vi "CMN_2DArr2Str.vi"(9 "separator":string=" ", 10 "array in":string[][](table)) -> (2 "string out":string)   [LabVIEW 2016]
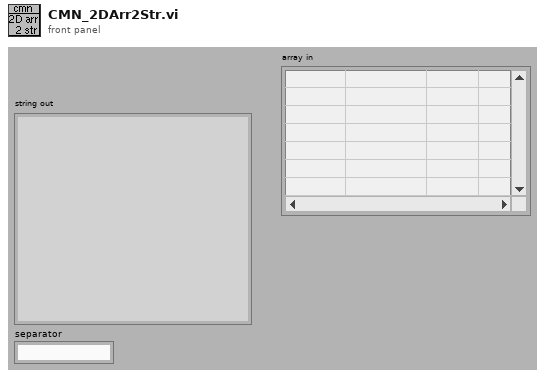
[diagram p1: front panel]
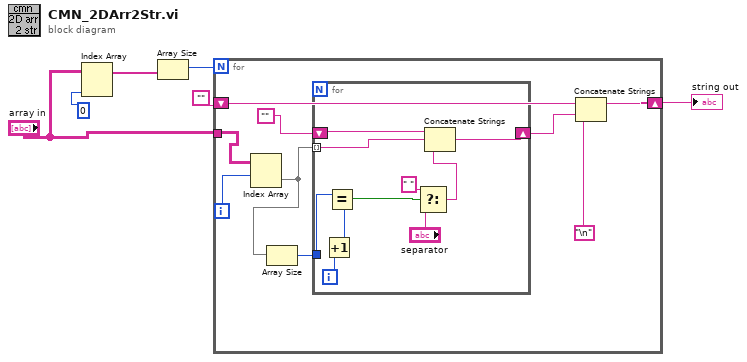
[diagram p0: block diagram]
diagram:
  n1 = Index Array(array="array in", index (col)=0) -> (element=w4:string[])  [unwired: 1 in]
  n2 = Array Size(array=w4) -> (size(s)=w2:i32)
  n3 = for {
    N: w2 -> [_]
    shift-right: [w15] -> w5
    shift-left: "" -> [w14]
    tunnel: "array in" -> [w11]
    i -> [w10]
    n4 = Index Array(array=w11, index (row)=w10) -> (element=w8:string[])  [unwired: 1 in]
    n5 = Array Size(array=w8) -> (size(s)=w7:i32)
    n6 = for {
      shift-right: [w25] -> w12
      shift-left: "" -> [w24]
      tunnel: w8 -> [w16] mode=indexing
      tunnel: w7 -> [w22]
      i -> [w23]
      n7 = Increment(x=w23) -> (x+1=w20:i32)
      n8 = Equal?(x=w22, y=w20) -> (x = y?=w21:bool)
      n9 = Select(t=" ", s=w21, f="separator") -> (s? t:f=w17:string)
      n10 = Concatenate Strings(w24, w16, w17) -> (w25:string)
    }
    n11 = Concatenate Strings(w14, w12, "\n") -> (w15:string)
  }
  "string out" <- w5
